vi "action_get_sub.vi"(0 "Thorlabs_OSA_64.lvclass:queue_action.ctlqueue ref":refnum<queue>, 11 "error":errorcluster) -> (4 "action":T1, 8 "action data":T2 {"par 4" format="%.2f"; "par 3" format="%.2f"; "par 2" format="%.2f"; "par" format="%.2f"}, 15 "error out":errorcluster)   [LabVIEW 2010, in "OSA.lvclass"]
uses:
  OSA.lvclass
  OSA20X_misc.lvlib
  typeDef/queue_action.ctl
  action_data.ctl
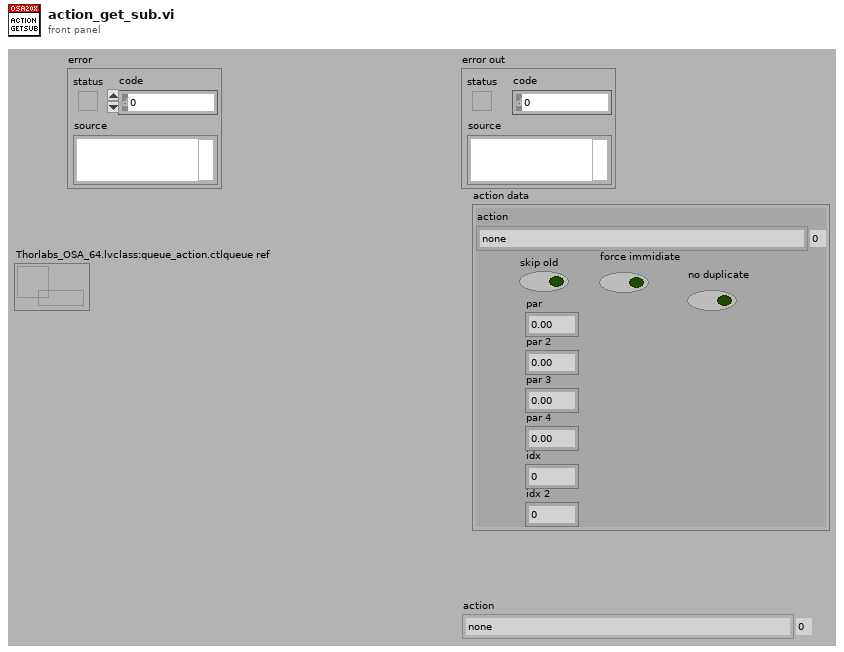
[diagram p1: front panel]
types:
  T1 = typedef "OSA.lvclass/queue_action.ctl" = enum16{"none", "stop", "GUI_plotInterferogram", "GUI_plotSpectrum", "GUI_plotInterferogramRescale", "GUI_plotSpectrumRescale", "GUI_plotInterferogramReset", "GUI_plotSpectrumReset", "GUI_plotInterferogramAutoScaleY", "GUI_plotSpectrumAutoScaleY", "GUI_plotInterferogramZoomOut", "GUI_plotSpectrumZoomOut", "GUI_plotInterferogramPane", "GUI_plotSpectrumPane", "GUI_plotInterferogramZoomMouse", "GUI_plotSpectrumZoomMouse", "ENVIRONMENT temperature", "ENVIRONMENT pressure", "MODE_resolution set", "MODE_resolution get", "MODE_sensitivity set", "MODE_sensitivity get", "MODE_PDTemperature set", "MODE_PDTemperature get", "REBOOT/RESET firmware", "ACQASYNC_acquireSingleSpectrum", "ACQASYNC_continuous start", "ACQASYNC_continuous stop\n", "ACQASYNC_get last interferogram", "ACQASYNC_get last spectrum", "ACQASYNC_get last waveNr", "ACQOPT_interferogram smoothing set", "ACQOPT_interferogram smoothing get", "ACQOPT_spectrum smoothing set", "ACQOPT_spectrum smoothing get", "ACQOPT_apodisation type set", "ACQOPT_apodisation type get", "ACQOPT_phase correction type set", "ACQOPT_phase correction type get", "ACQOPT_acqIntervall_set", "ACQOPT_acqIntervall_get", "ACQOPT_average spectrum set", "ACQOPT_average spectrum get", "ACQOPT_rolling average set", "ACQOPT_rolling average get", "ACQOPT_zero fill factor set", "ACQOPT_zero fill factor get", "ACQOPT_cycle counting set", "ACQOPT_cycle counting get", "ACQOPT_air measure option set", "ACQOPT_air measure option get", "ACQOPT_gainLevel auto get", "ACQOPT_gainLevel auto set", "ACQOPT_gainLevel get", "ACQOPT_gainLevel set", "ACQOPT_getAll", "INSTRUMENT_PROPERTY_range_WaveNr_min", "INSTRUMENT_PROPERTY_range_WaveNr_max", "INSTRUMENT_PROPERTY_reference_wavelength_cm^-1", "INSTRUMENT_PROPERTY_samplesPerRefPeriod", "INSTRUMENT_PROPERTY_resolution_waveNrPercm", "INSTRUMENT_PROPERTY_availableGainLevels", "INSTRUMENT_PROPERTY_status", "CONVERT", "ANALYSE_POWER", "ANALYSE_PEAKS", "ANALYSE_WAVELENGTH", "ANALYSE_SPECTRUM", "ANALYSE_INTERFEROGRAM", "ANALYSE_COHERENCE_LENGTH", "MATH", "MATH_power", "MATH_peaks", "FILE", "miscellaneous"}
  T2 = typedef "OSA.lvclass/action_data.ctl" = cluster{"action":T1, "skip old":bool, "force immidiate":bool, "par":dbl, "par 2":dbl, "par 3":dbl, "par 4":dbl, "idx":i32, "idx 2":i32, "no duplicate":bool}
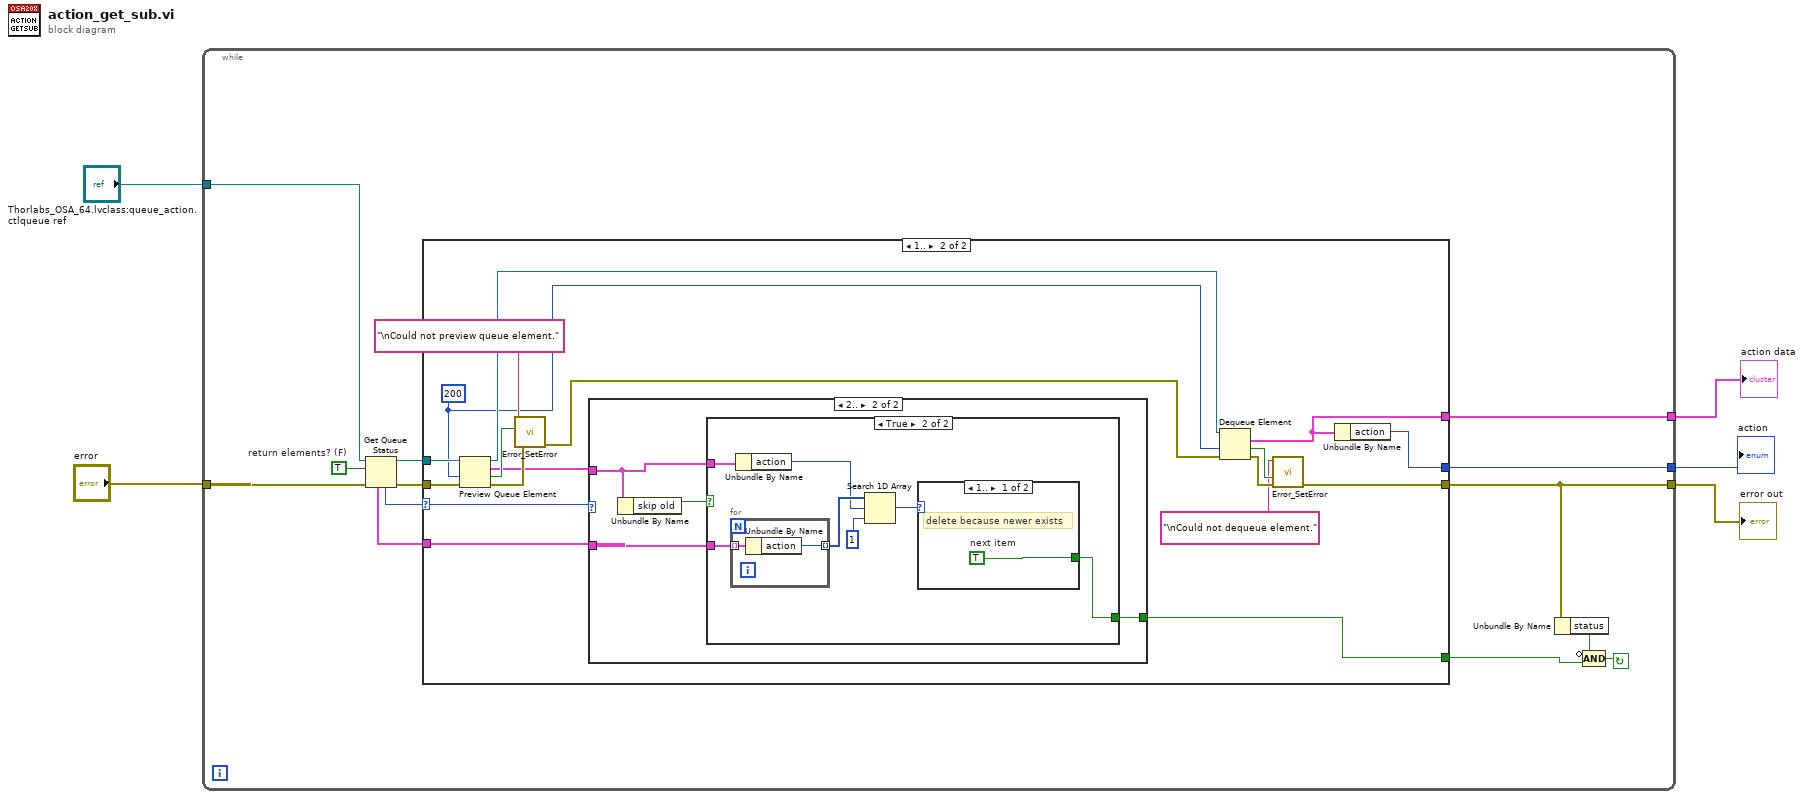
[diagram p0: block diagram]
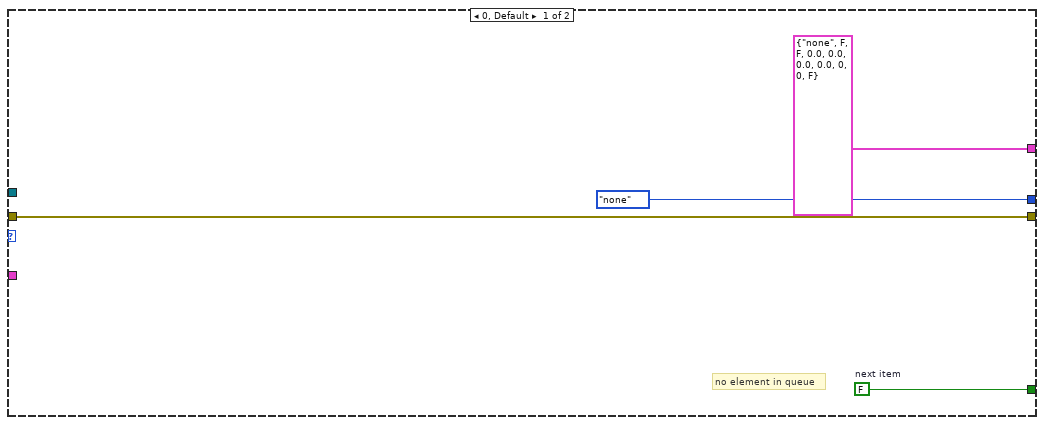
[diagram p2: hidden frame]
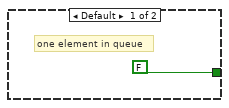
[diagram p3: hidden frame]
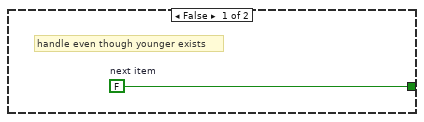
[diagram p4: hidden frame]
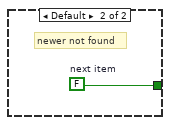
[diagram p5: hidden frame]
diagram:
  n1 = while {
    tunnel: "error" -> [w18]
    tunnel: [w12] -> w2
    tunnel: [w11] -> w3
    tunnel: [w10] -> w4
    tunnel: "Thorlabs_OSA_64.lvclass:queue_action.ctlqueue ref" -> [w6]
    stop <- w9 continue-if-true
    w17 = TRUE  # return elements? (F)
    n2 = Get Queue Status(queue=w6, return elements? (F)=w17, error in (no error)=w18) -> (queue out=w13:refnum<queue>, error out=w14:errorcluster, # elements in queue=w16:i32, elements=w15:T2[])  [unwired: 4 out]
    n3 = case shown="1.." w16 {
      selector: w16 -> [_ w37]
      tunnel: w15 -> [_ w38]
      tunnel: w14 -> [w21 w40]
      tunnel: w13 -> [_ w39]
      tunnel: [queue_action."none" ("action") w29] -> w12
      tunnel: [T2 {"action"=enum."none", "skip old"=FALSE, "force immidiate"=FALSE, "par"=0.0, "par 2"=0.0, "par 3"=0.0, "par 4"=0.0, "idx"=0, "idx 2"=0, "no duplicate"=FALSE} ("action data") w23] -> w11
      tunnel: [w21 w30] -> w10
      tunnel: [w20 w36] -> w7
      frame 0, Default {
        w20 = FALSE  # next item
        # "no element in queue"
      }
      frame 1.. {
        w25 = 200 ("timeout in ms (-1)")
        n4 = Preview Queue Element(queue=w39, timeout in ms (-1)=w25, error in (no error)=w40) -> (queue out=w26:refnum<queue>, element=w32:T2, timed out?=w34:bool, error out=w35:errorcluster)
        n5 = call "Error_SetError.vi"("error in"=w35, "status (true)"=w34, "source(\"\")"="\nCould not preview queue element." ("source(\"\")")) -> ("error out"=w24:errorcluster)  [unwired: 4 in]
        n6 = case shown="2.." w37 {
          tunnel: w38 -> [_ w45]
          tunnel: w32 -> [_ w42]
          tunnel: [FALSE w43] -> w36
          frame Default {
            # "one element in queue"
          }
          frame 2.. {
            n7 = Unbundle By Name(w42) -> ("skip old"=w44:bool)
            n8 = case shown="True" w44 {
              tunnel: w45 -> [_ w53]
              tunnel: w42 -> [_ w50]
              tunnel: [w46 w49] -> w43
              frame False {
                w46 = FALSE  # next item
                # "handle even though younger exists"
              }
              frame True {
                n9 = for {
                  tunnel: w53 -> [w57] mode=indexing
                  tunnel: [w56] -> w52 mode=indexing
                  n10 = Unbundle By Name(w57) -> ("action"=w56:T1)
                }
                n11 = Unbundle By Name(w50) -> ("action"=w51:T1)
                n12 = Search 1D Array(1D array=w52, element=w51, start index (0)=1) -> (index of element=w48:i32)
                n13 = case shown="1.." w48 {
                  tunnel: [w54 w55] -> w49
                  frame 1.. {
                    w54 = TRUE  # next item
                    # "delete because newer exists"
                  }
                  frame Default {
                    w55 = FALSE  # next item
                    # "newer not found"
                  }
                }
              }
            }
          }
        }
        n14 = Dequeue Element(queue=w26, timeout in ms (-1)=w25, error in (no error)=w24) -> (element=w23:T2, timed out?=w31:bool, error out=w28:errorcluster)  [unwired: 1 out]
        n15 = call "Error_SetError.vi"("error in"=w28, "status (true)"=w31, "source(\"\")"="\nCould not dequeue element." ("source(\"\")")) -> ("error out"=w30:errorcluster)  [unwired: 4 in]
        n16 = Unbundle By Name(w23) -> ("action"=w29:T1)
      }
    }
    n17 = Unbundle By Name(w10) -> ("status"=w8:bool)
    n18 = Compound Arithmetic op=AND(invert w8, w7) -> (w9:bool)
  }
  "error out" <- w4
  "action data" <- w3
  "action" <- w2
